vi "lvssh2_userauth_keyboard_interactive_response_function_handler_32.vi"(9 "lvssh2_userauth_keyboard_interactive_response_function":refnum<vi>, 10 "Stop Event Ref":refnum<user-event>, 11 "User Event Ref":refnum<user-event>) -> ()   [LabVIEW 2017, in "libssh2.lvlib"]
uses:
  libssh2.lvlib
  lvssh2_userauth_keyboard_interactive_response_function_input_args_32.ctl
  lvssh2_userauth_keyboard_interactive_prompt.ctl
  lvssh2_extensions_64.dll
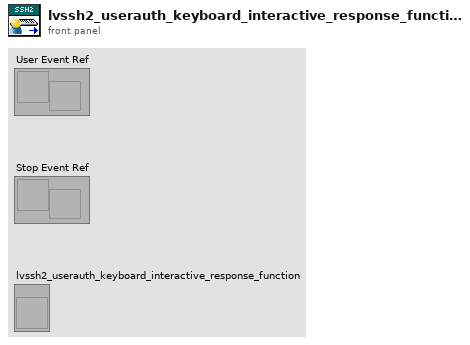
[diagram p1: front panel]
types:
  T1 = typedef "libssh2.lvlib/lvssh2_userauth_keyboard_interactive_prompt.ctl" = cluster{"text":string, "echo":bool}
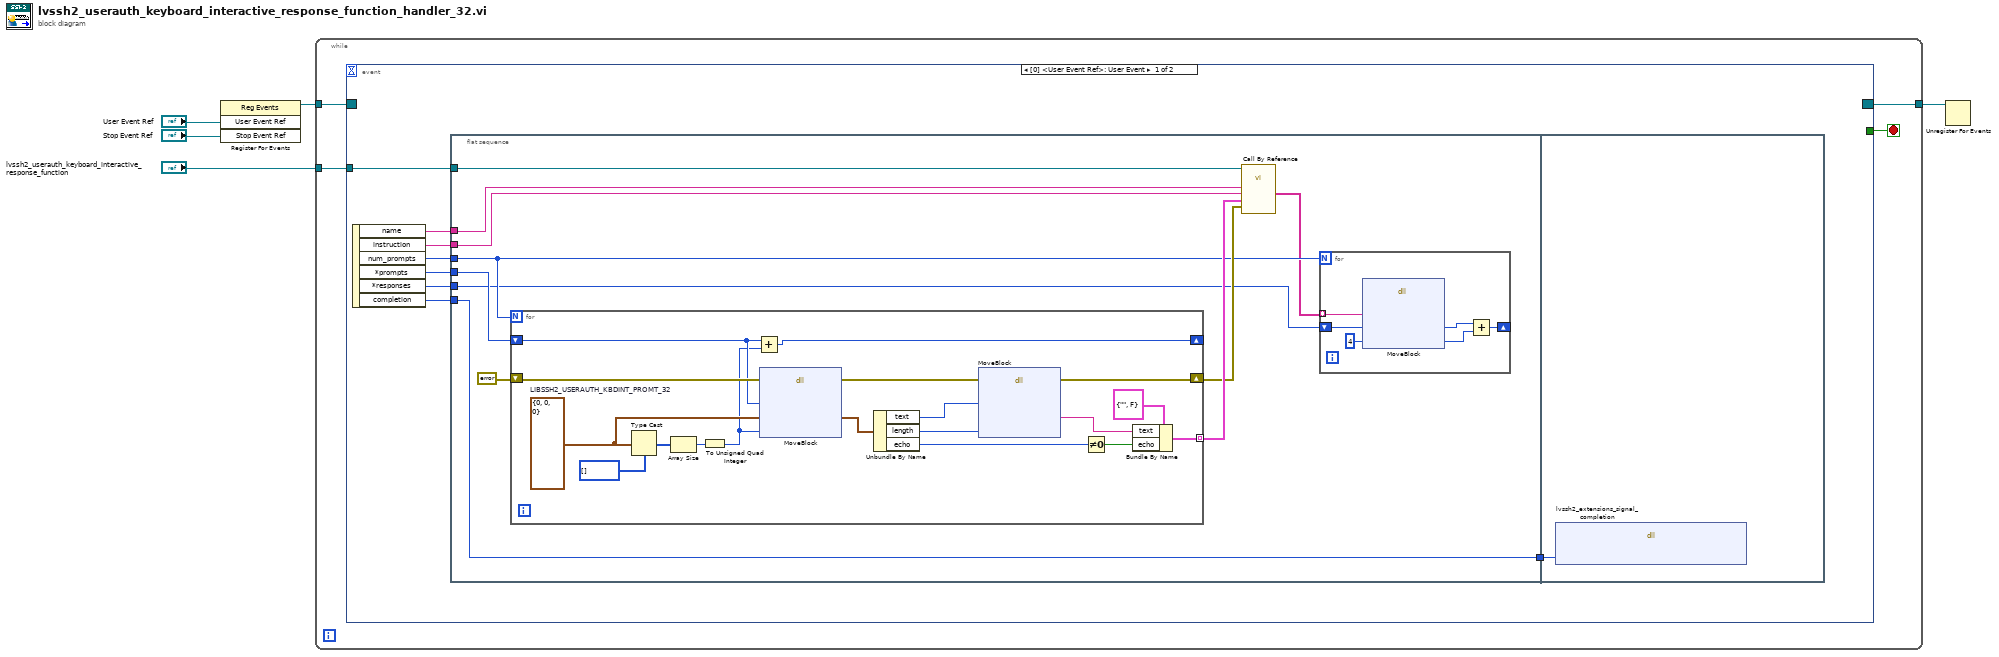
[diagram p0: block diagram]
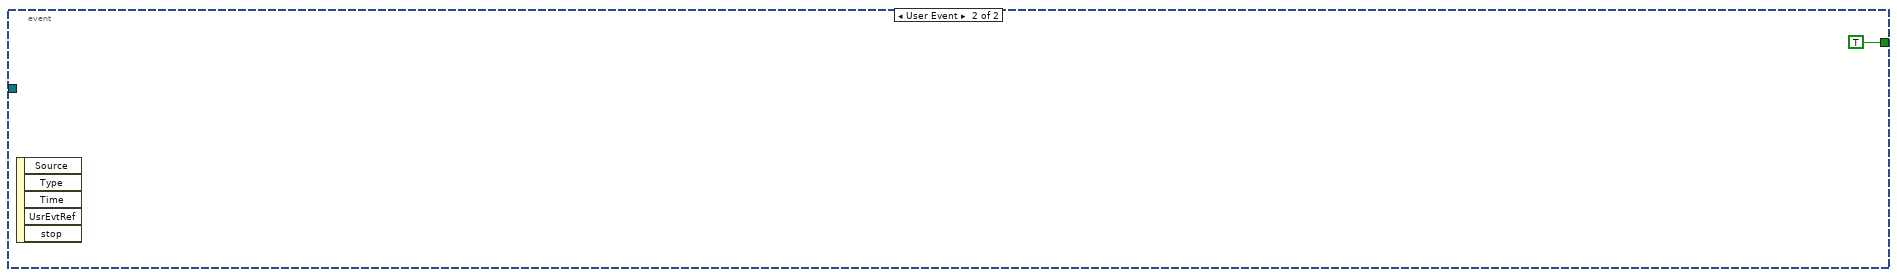
[diagram p2: hidden frame]
diagram:
  n1 = register-events("User Event Ref", "Stop Event Ref") -> (reference out=w4:refnum<event-registration>)  [unwired: 2 in, 1 out]
  n2 = while {
    tunnel: "lvssh2_userauth_keyboard_interactive_response_function" -> [w9]
    tunnel: w4 -> [w8]
    tunnel: [w7] -> w1
    stop <- w6 stop-if-true
    n3 = event shown="[0] <User Event Ref>: User Event" {
      selector: w8 -> [_ _]
      dyn-events: [_ _] -> w7
      timeout: _ -> [_ _]
      tunnel: w9 -> [w16 _]
      tunnel: [_ TRUE] -> w6
      event User Event {
        n4 = event-data() -> ("name"=w15:string, "instruction"=w14:string, "num_prompts"=w13:i32, "*prompts"=w12:u32, "*responses"=w11:u32, "completion"=w10:u32)  [unwired: 1 in]
        n5 = flat-sequence {
          tunnel: w16 -> [w28]
          tunnel: w15 -> [w27]
          tunnel: w14 -> [w26]
          tunnel: w12 -> [w25]
          tunnel: w13 -> [w21]
          tunnel: w11 -> [w19]
          tunnel: w10 -> [w18]
          tunnel: [w18] -> w17
          tunnel: w17 -> [w53]
          frame #0 {
            n6 = for {
              N: w21 -> [_]
              tunnel: [w41] -> w24 mode=indexing
              shift-right: [w40] -> _
              shift-left: w25 -> [w37]
              shift-right: [w39] -> w23
              shift-left: errorcluster {"status"=FALSE, "code"=0, "source"=""} ("error out") -> [w38]
              w52 = cluster{"text":u32, "length":u32, "echo":u8} {"text"=0, "length"=0, "echo"=0}  # LIBSSH2_USERAUTH_KBDINT_PROMT_32
              n7 = Type Cast(type=u8[] [], x=w52) -> (*(type *) &x=w50:u8[])
              n8 = Array Size(array=w50) -> (size(s)=w36:i32)
              n9 = To Unsigned Quad Integer(1:w36) -> (0:w35:u64)
              n10 = Add(x=w37, y=w35) -> (x+y=w40:u64)
              n11 = dll-call lib="LabVIEW" fn="MoveBlock"(error in=w38, "ps"=w37, "pd"=w52, "size"=w35) -> (error out=w49:errorcluster, "pd"=w48:cluster{"text":u32, "length":u32, "echo":u8})  [unwired: 5 in, 1 out]
              n12 = Unbundle By Name(w48) -> ("text"=w47:u32, "length"=w46:u32, "echo"=w43:u8)
              n13 = dll-call lib="LabVIEW" fn="MoveBlock"(error in=w49, "ps"=w47, "size"=w46) -> (error out=w39:errorcluster, "pd"=w44:string)  [unwired: 6 in, 1 out]
              n14 = Not Equal To 0?(x=w43) -> (x != 0?=w42:bool)
              n15 = Bundle By Name(cluster=T1 {"text"="", "echo"=FALSE} ("prompt"), "text"=w44, "echo"=w42) -> (w41:T1)
            }
            n16 = call-by-ref "?"(reference=w28, "error in (no error)"=w23, "prompts"=w24, "instruction"=w26, "name"=w27) -> ("responses"=w20:string[])  [unwired: 7 in, 3 out]
            n17 = for {
              N: w21 -> [_]
              tunnel: w20 -> [w32] mode=indexing
              shift-right: [w30] -> _
              shift-left: w19 -> [w33]
              n18 = dll-call lib="LabVIEW" fn="MoveBlock"("ps"=w32, "pd"=w33, "size"=u64 4) -> ("pd"=w31:u64, "size"=w29:u64)  [unwired: 5 in, 2 out]
              n19 = Add(x=w31, y=w29) -> (x+y=w30:u64)
            }
          }
          frame #1 {
            n20 = dll-call lib="C:/Users/Pascal/Projects/Home/lvssh2/libssh2/lvssh2_extensions**.*" fn="lvssh2_extensions_signal_completion"("completion"=w53) -> ()  [unwired: 5 in, 2 out]
          }
        }
      }
      event User Event {
        n21 = event-data() -> ()  [unwired: 1 in, 5 out]
      }
    }
  }
  n22 = Unregister For Events(event registration refnum=w1) -> ()  [unwired: 1 in, 1 out]
